vi "TDMS_Viewer_Simple.vi"() -> ()   [LabVIEW 2022 SP3]
uses:
  <vilib>/Utility/TDMS File Viewer/NI_TDMS File Viewer.lvlib
panel:
  in  "file in":path=path "C:/Users/LAV-UFSC/OneDrive - UFSC/Documents-LAV-UFSC/LAV-TCC/Dados-Experimentos/Dados-Bancada-LABVIEW/07-Jul-23_5-09-18-PM.tdms"
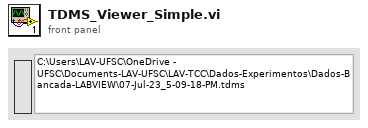
[diagram p1: front panel]
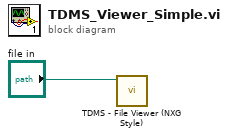
[diagram p0: block diagram]
diagram:
  n1 = call <vilib>:"TDMS - File Viewer (NXG Style).vi"("file in"="file in") -> ()  [unwired: 9 in, 2 out]
